vi "LV to ITX 2.2 2D w X&Y.vi"(0 "Commands":string, 1 "Kill X&Y waves?":bool=TRUE, 4 "Y Array name":string, 5 "filename":path, 6 "Y 1D Array":dbl[](array[numeric]), 7 "Notes":string, 8 "X  Array name":string, 9 "X 1D Array":dbl[](array[numeric]), 10 "2D Array name":string, 11 "2D Array":dbl[][](array[numeric])) -> (3 "file":path)   [LabVIEW 2013]
panel:
  out "String 2":string
  out "String":string
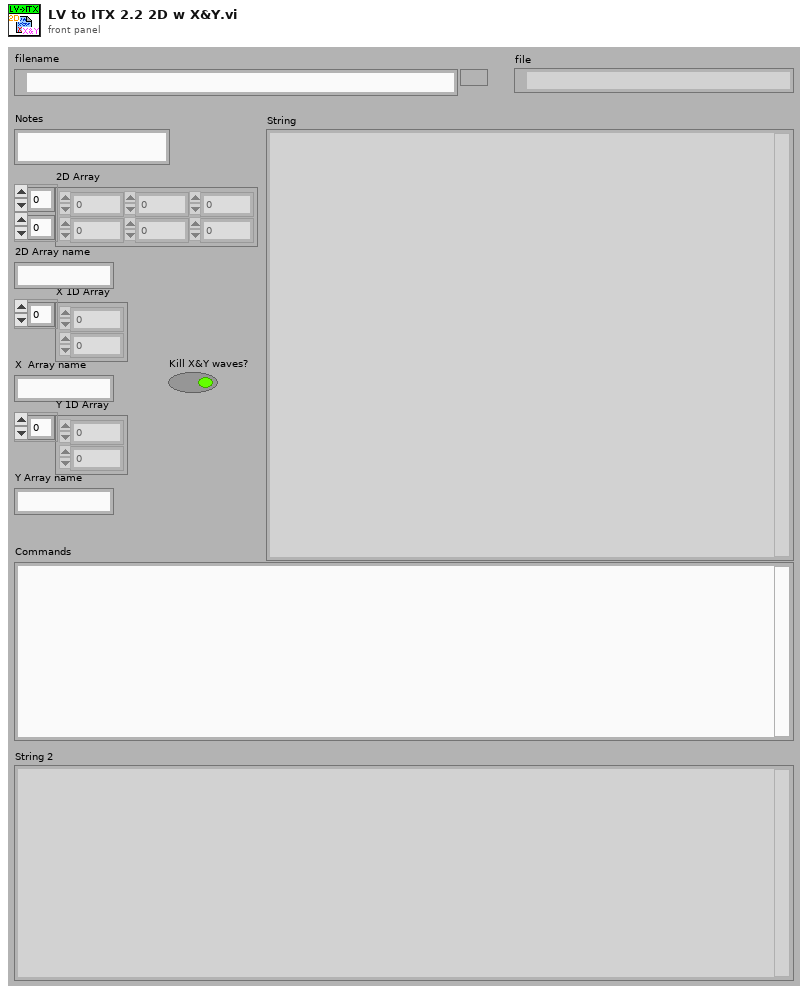
[diagram p1: front panel]
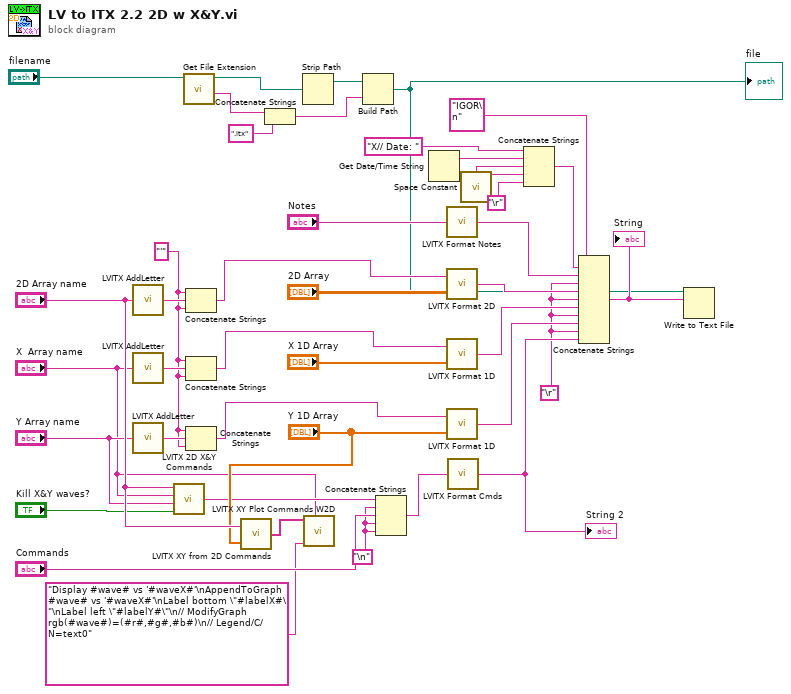
[diagram p0: block diagram]
diagram:
  w15 = "'" ("string")
  w1 = "\n"
  w29 = "\r"
  n1 = call "LVITX AddLetter.vi"("String"="2D Array name") -> ("output string"=w18:string)
  n2 = call "LVITX AddLetter.vi"("String"="X  Array name") -> ("output string"=w17:string)
  n3 = call "LVITX AddLetter.vi"("String"="Y Array name") -> ("output string"=w16:string)
  n4 = call "LVITX 2D X&Y Commands.vi"("Kill X&Y waves?"="Kill X&Y waves?", "Y wave"="Y Array name", "X wave"="X  Array name", "2D wave"="2D Array name") -> ("result string"=w8:string)
  n5 = call <vilib>:"Get File Extension.vi"("file"="filename") -> ("filename without extension"=w25:string, "dup file"=w22:path)  [unwired: 1 in, 8 out]
  n6 = Concatenate Strings(w15, w18, w15) -> (w12:string)
  n7 = Concatenate Strings(w15, w17, w15) -> (w13:string)
  n8 = Concatenate Strings(w15, w16, w15) -> (w14:string)
  n9 = call "LVITX XY from 2D Commands.vi"("Y 1D Array"="Y 1D Array", "2D wave"="2D Array name") -> ("wavenames"=w5:string[])
  n10 = Concatenate Strings(w25, ".itx") -> (w20:string)
  n11 = Strip Path(path=w22) -> (stripped path=w21:path)  [unwired: 1 out]
  n12 = call "LVITX XY Plot Commands W2D.vi"("wavenames"=w5, "input string"="Display #wave# vs '#waveX#'\nAppendToGraph #wave# vs '#waveX#'\nLabel bottom \"#labelX#\"\nLabel left \"#labelY#\"\n// ModifyGraph rgb(#wave#)=(#r#,#g#,#b#)\n// Legend/C/N=text0", "X wave"="X  Array name") -> ()  [unwired: 2 in, 1 out]
  n13 = Build Path(base path=w21, name or relative path=w20) -> (appended path=w2:path)
  "file" <- w2
  n14 = Concatenate Strings(w8, w1, "Commands", w1, w1) -> (w23:string)
  n15 = Get Date/Time String() -> (date string=w40:string, time string=w41:string)  [unwired: 3 out]
  n16 = call "LVITX Format Notes.vi"("Notes"="Notes") -> ("String"=w30:string)
  n17 = call "LVITX Format 2D.vi"("2D Array"="2D Array", "2D Array name"=w12) -> ("String"=w34:string)
  n18 = call "LVITX Format 1D.vi"("X 1D Array"="X 1D Array", "X  Array name"=w13) -> ("String"=w33:string)
  n19 = call "LVITX Format 1D.vi"("X 1D Array"="Y 1D Array", "X  Array name"=w14) -> ("String"=w32:string)
  n20 = call "LVITX Format Cmds.vi"("Commands"=w23) -> ("String"=w31:string)
  "String 2" <- w31
  n21 = call <vilib>:"Space Constant.vi"() -> ("String"=w27:string)
  n22 = Concatenate Strings("X// Date: " ("format string"), w40, w27, w41, "\r") -> (w39:string)
  n23 = Concatenate Strings("IGOR\n", w39, w30, w29, w34, w29, w33, w29, w32, w29, w31) -> (w28:string)
  "String" <- w28
  n24 = Write to Text File(file (use dialog)=w2, text=w28) -> ()  [unwired: 1 in, 4 out]
